vi "FMV - click.vi"(8 "error in (no error)":errorcluster, 11 "JSON string":string) -> (0 "error out":errorcluster, 3 "value":string)   [LabVIEW 2020, in "ui-testing.lvlib"]
doc: "copyright: Thomas Zilliox©"
uses:
  ui-testing.lvlib
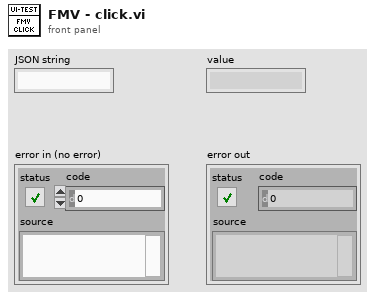
[diagram p1: front panel]
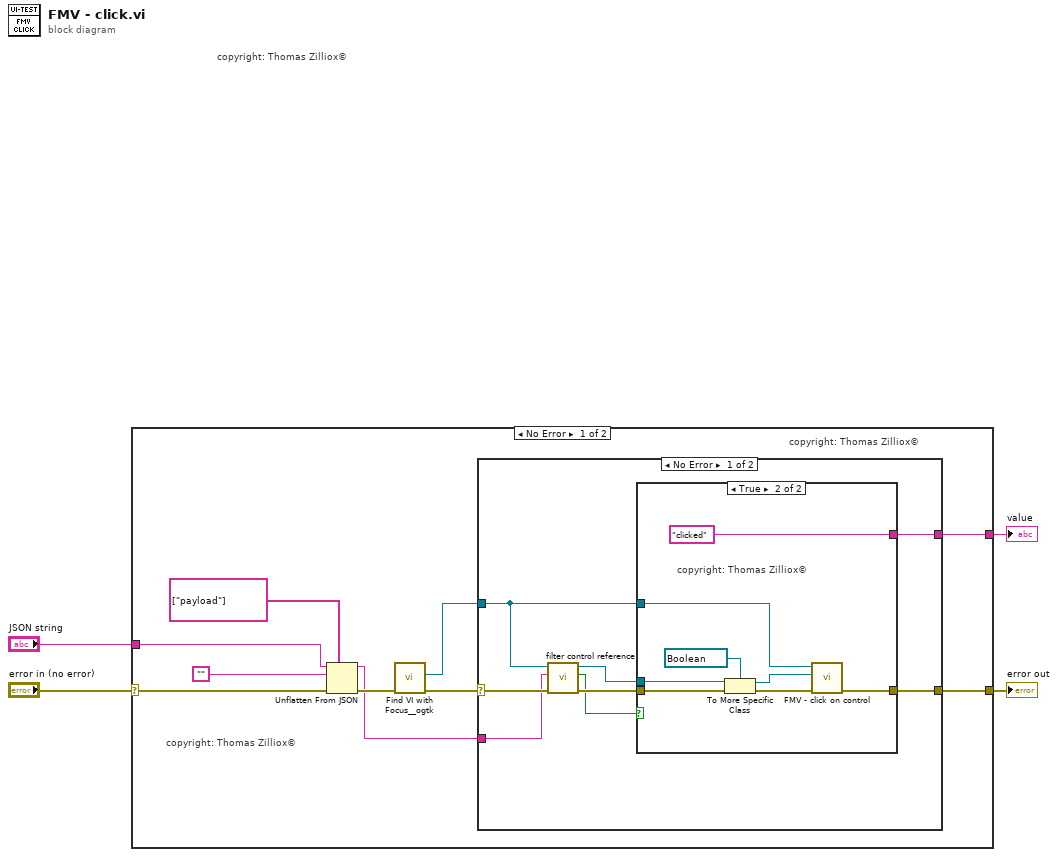
[diagram p0: block diagram]
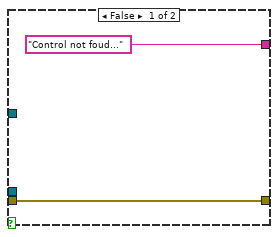
[diagram p2: hidden frame]
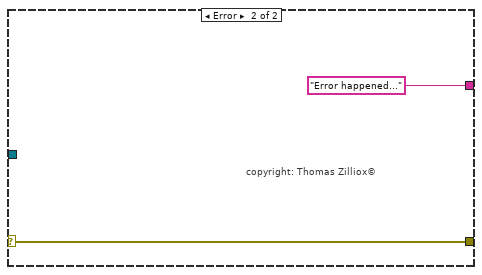
[diagram p3: hidden frame]
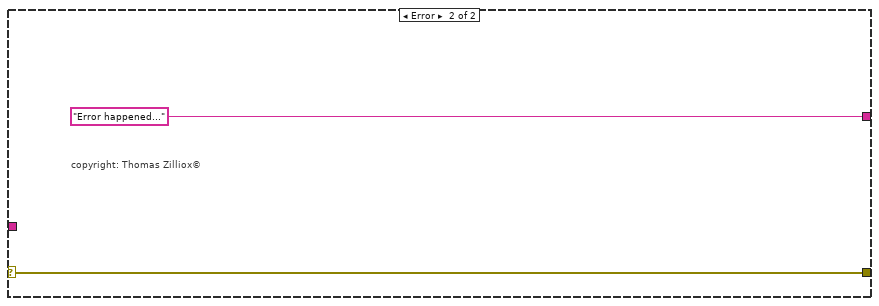
[diagram p4: hidden frame]
diagram:
  # "copyright: Thomas Zilliox©"
  n1 = case shown="No Error" "error in (no error)" {
    selector: "error in (no error)" -> [w12 w36]
    tunnel: [w5 w36] -> w3
    tunnel: "JSON string" -> [w11 _]
    tunnel: [w7 "Error happened..."] -> w1
    frame No Error {
      # "copyright: Thomas Zilliox©"
      # "copyright: Thomas Zilliox©"
      n2 = Unflatten From JSON(path=string[] ["payload"], JSON string=w11, type and defaults="", error in (no error)=w12) -> (value=w8:string, error out=w13:errorcluster)  [unwired: 3 in]
      n3 = call <userlib>:"Find VI with Focus__ogtk.vi"("error in"=w13) -> ("error out"=w6:errorcluster, "VI with Focus"=w9:refnum<vi>)  [unwired: 6 in, 3 out]
      n4 = case shown="No Error" w6 {
        selector: w6 -> [w21 w34]
        tunnel: [w19 w34] -> w5
        tunnel: w8 -> [w20 _]
        tunnel: [w16 "Error happened..."] -> w7
        tunnel: w9 -> [w15 _]
        frame No Error {
          n5 = call "filter control reference.vi"("error in (no error)"=w21, "Control label"=w20, "VI (Caller)"=w15) -> ("error out"=w18:errorcluster, "Control found"=w17:bool, "Control ref"=w22:refnum<vi>)  [unwired: 6 in]
          n6 = case shown="True" w17 {
            tunnel: w22 -> [_ w32]
            tunnel: w15 -> [_ w29]
            tunnel: [w23 w28] -> w19
            tunnel: w18 -> [w23 w27]
            tunnel: ["Control not foud..." "clicked" ("VI Name")] -> w16
            frame False {
            }
            frame True {
              # "copyright: Thomas Zilliox©"
              n7 = To More Specific Class(target class=refnum<vi> refnum ("Reference to Button"), reference=w32, error in=w27) -> (specific class reference=w30:refnum<vi>, error out=w26:errorcluster)
              n8 = call "FMV - click on control.vi"("error in (no error)"=w26, "Reference to Button"=w30, "VI Reference"=w29) -> ("error out"=w28:errorcluster)  [unwired: 8 in]
            }
          }
        }
        frame Error {
          # "copyright: Thomas Zilliox©"
        }
      }
    }
    frame Error {
      # "copyright: Thomas Zilliox©"
    }
  }
  "error out" <- w3
  "value" <- w1
